vi "Config Get Key Names.vi"(7 "Section Name":string, 8 "error in":errorcluster, 11 "Config Cluster in":T1) -> (0 "error out":errorcluster, 1 "Key Array":string[](array[string]), 2 "Found?":bool, 3 "Config Cluster out":T1)   [LabVIEW 2017]
uses:
  Config Cluster.ctl
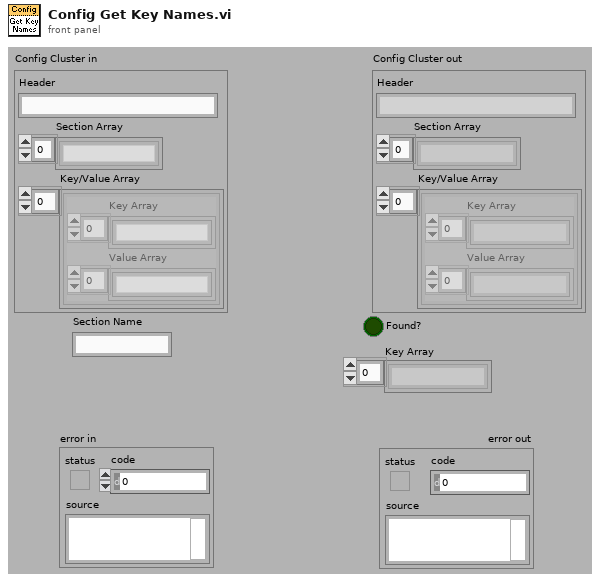
[diagram p1: front panel]
types:
  T1 = typedef "Config Cluster.ctl" = cluster{"Header":string, "Section Array":string[], "Key/Value Array":cluster{"Key Array":string[], "Value Array":string[]}[]}
  T2 = cluster{"Key Array":string[], "Value Array":string[]}[]
  T3 = cluster{"Key Array":string[], "Value Array":string[]}
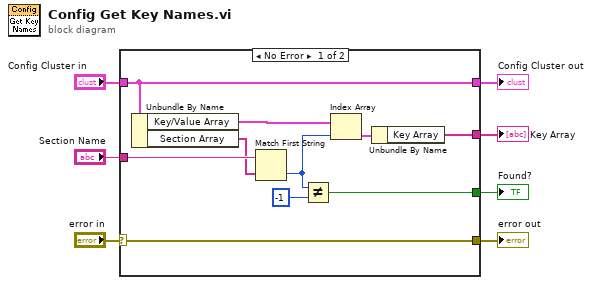
[diagram p0: block diagram]
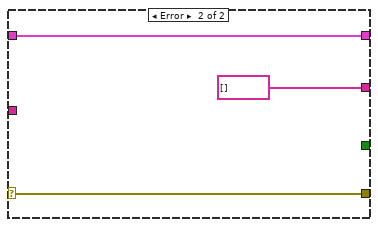
[diagram p2: hidden frame]
diagram:
  n1 = case shown="No Error" "error in" {
    selector: "error in" -> [w14 w19]
    tunnel: [w14 w19] -> w6
    tunnel: "Config Cluster in" -> [w17 w20]
    tunnel: [w17 w20] -> w4
    tunnel: "Section Name" -> [w16 _]
    tunnel: [w11 string[] [] ("Key Array")] -> w2
    tunnel: [w8 _] -> w1
    frame No Error {
      n2 = Unbundle By Name(w17) -> ("Key/Value Array"=w13:T2, "Section Array"=w10:string[])
      n3 = Match First String(2:w10, 3:w16) -> (0:w12:i32)  [unwired: 1 out]
      n4 = Not Equal?(x=w12, y=-1) -> (x != y?=w8:bool)
      n5 = Index Array(array=w13, index=w12) -> (element=w9:T3)
      n6 = Unbundle By Name(w9) -> ("Key Array"=w11:string[])
    }
    frame Error {
    }
  }
  "error out" <- w6
  "Config Cluster out" <- w4
  "Key Array" <- w2
  "Found?" <- w1
